vi "GPIB_autodetect.vi"(7 "ID command":string, 8 "error in (no error)":errorcluster, 9 "Verify GPIB address":bool, 10 "Instrument address in":refnum<visa-resource-name>, 11 "InstrControl in":refnum<class "InstrControl.lvclass">) -> (0 "error out":errorcluster, 2 "Instrument address out":refnum<visa-resource-name>, 3 "InstrControl out":refnum<class "InstrControl.lvclass">)   [LabVIEW 2013, in "InstrControl.lvclass"]
uses:
  InstrControl.lvclass
panel:
  out "addresses found":string[](array[string])
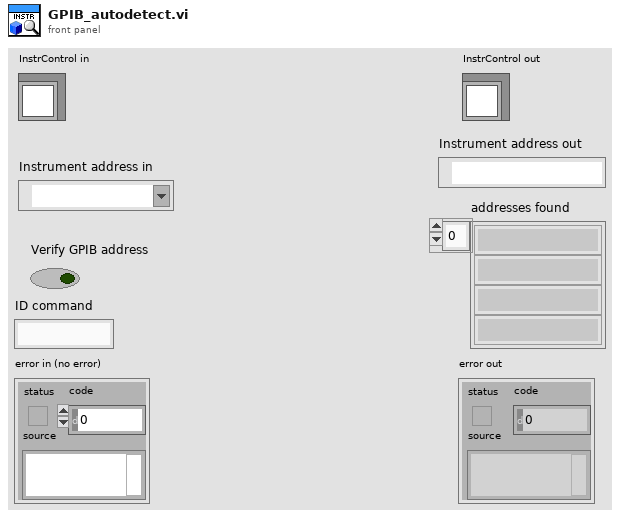
[diagram p1: front panel]
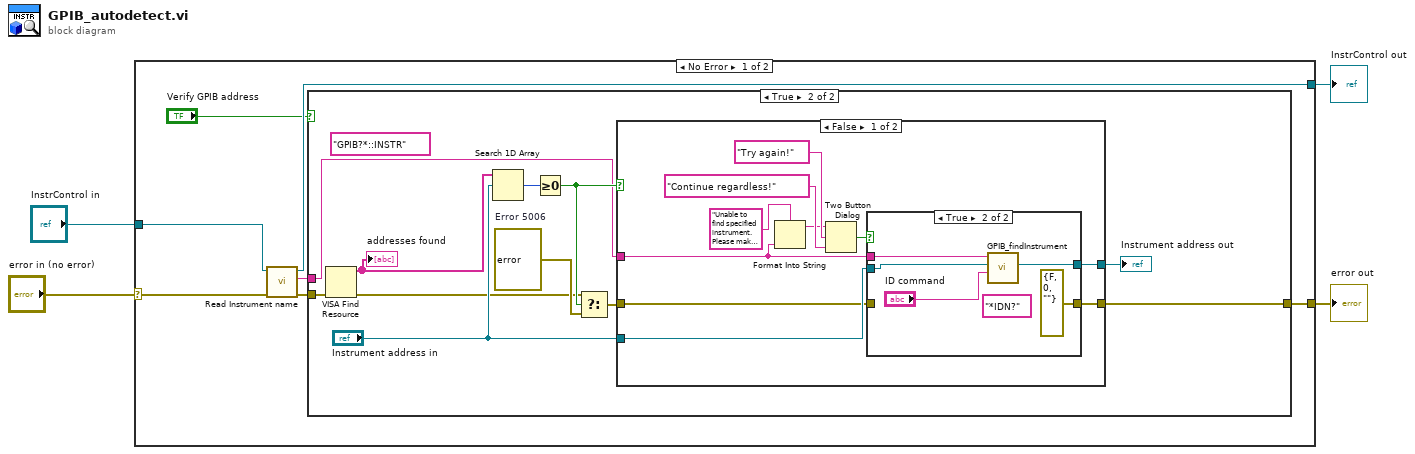
[diagram p0: block diagram]
diagram:
  n1 = case shown="No Error" "error in (no error)" {
    selector: "error in (no error)" -> [w10 w44]
    tunnel: [w7 w44] -> w3
    tunnel: [w9 w43] -> w1
    tunnel: "InstrControl in" -> [w11 w43]
    frame No Error {
      n2 = call-dynamic "Read Instrument name.vi"("error in (no error)"=w10, "InstControl in"=w11) -> ("error out"=w8:errorcluster, "Instrument name"=w6:string, "InstControl out"=w9:refnum<class "InstrControl.lvclass">)  [unwired: 7 in]
      n3 = case shown="True" "Verify GPIB address" {
        tunnel: w8 -> [w12 w22]
        tunnel: [w12 w16] -> w7
        tunnel: w6 -> [_ w15]
        frame False {
        }
        frame True {
          w23 = errorcluster {"status"=FALSE, "code"=5005, "source"="Unable to find specified instrument.  Please make sure the it is connected to your system and switched on."}  # Error 5006
          (unwired) "GPIB?*::INSTR" ("expression (\"\")")
          n4 = VISA Find Resource(8:w22) -> (0:w13:errorcluster, 3:w14:string[])  [unwired: 2 in, 1 out]
          "addresses found" <- w14
          n5 = Search 1D Array(1D array=w14, element="Instrument address in") -> (index of element=w20:i32)  [unwired: 1 in]
          n6 = Greater Or Equal To 0?(x=w20) -> (x >= 0?=w19:bool)
          n7 = Select(t=w13, s=w19, f=w23) -> (s? t:f=w17:errorcluster)
          n8 = case shown="False" w19 {
            tunnel: "Instrument address in" -> [w30 w42]
            tunnel: [w29 w42] -> w21
            tunnel: w17 -> [w28 w41]
            tunnel: [w27 w41] -> w16
            tunnel: w15 -> [w25 _]
            frame False {
              n9 = Format Into String(format string="Unable to find specified instrument.  Please make sure the it is connected to your system and switched on.\n\n%s" ("source"), w25) -> (resulting string=w24:string)  [unwired: 2 in, 1 out]
              n10 = Two Button Dialog(message=w24, 1:"Continue regardless!", 2:"Try again!") -> (T button?=w31:bool)
              n11 = case shown="True" w31 {
                tunnel: w30 -> [w35 w40]
                tunnel: [w35 w39] -> w29
                tunnel: w28 -> [w34 _]
                tunnel: [w34 errorcluster {"status"=FALSE, "code"=0, "source"=""} ("error constant")] -> w27
                tunnel: w25 -> [_ w37]
                frame False {
                }
                frame True {
                  (unwired) "*IDN?" ("regular expression")
                  n12 = call "GPIB_findInstrument.vi"("ID command"="ID command", "revised Instrument address"=w40, "Instrument name IN"=w37) -> ("revised GPIB address OUT"=w39:refnum<visa-resource-name>)  [unwired: 8 in]
                }
              }
            }
            frame True {
            }
          }
          "Instrument address out" <- w21
        }
      }
    }
    frame Error {
    }
  }
  "error out" <- w3
  "InstrControl out" <- w1
